vi "Camdefocused.vi"() -> ()   [LabVIEW 2011]
panel:
  out "CamDefocussed":bool
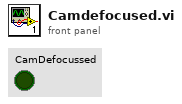
[diagram p1: front panel]
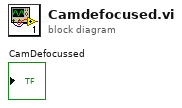
[diagram p0: block diagram]
diagram:
